vi "Distance Step Counter.vi"(8 "Distance (in)":dbl=40.0 format="%#_13g", 9 "Base Step":i32, 10 "Step":i32, 11 "RobotDriveDevRef":T1) -> (1 "Progress":dbl, 2 "Finished?":bool, 3 "Step out":i32)   [LabVIEW 2016]
uses:
  <vilib>/Rock Robotics/WPI/RobotDrive/WPI_RobotDriveDevRef.ctl
  <vilib>/Rock Robotics/WPI/MotorControl/WPI_MotorControlDeviceRef.ctl
  <vilib>/Rock Robotics/WPI/MotorControl/WPI_MotorControlType.ctl
  <vilib>/Rock Robotics/SystemInterfaces/DIO/FPGA_DIOPWMChannel.ctl
  <vilib>/Rock Robotics/WPI/PWM/WPI_PWMDeadband.ctl
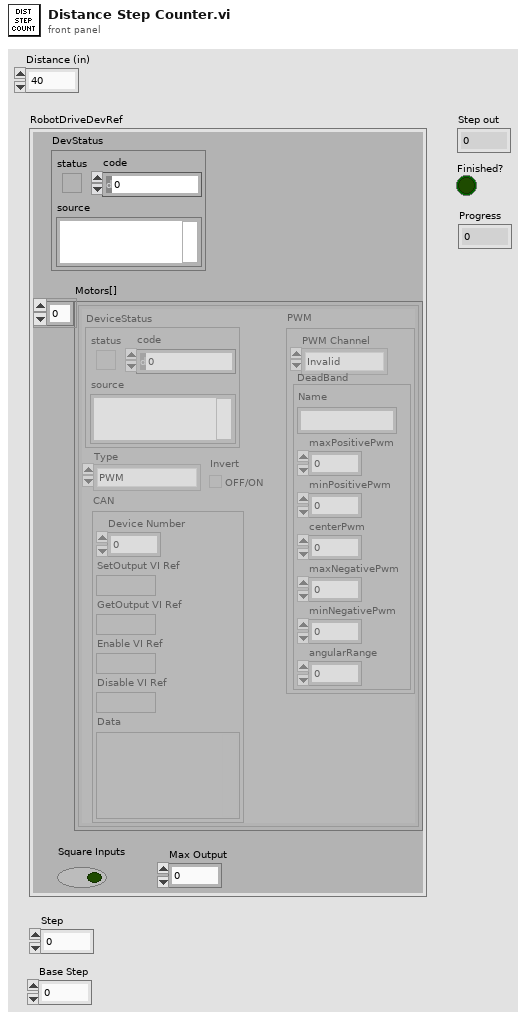
[diagram p1: front panel]
types:
  T1 = typedef "WPI_RobotDriveDevRef.ctl" = cluster{"DevStatus":errorcluster, "Motors[]":T2[], "Square Inputs":bool, "Max Output":dbl}
  T2 = typedef "WPI_MotorControlDeviceRef.ctl" = cluster{"DeviceStatus":errorcluster, "Type":T3, "PWM":cluster{"PWM Channel":T4, "DeadBand":T5}, "CAN":cluster{"Device Number":u8, "SetOutput VI Ref":variant, "GetOutput VI Ref":variant, "Enable VI Ref":variant, "Disable VI Ref":variant, "Data":variant}, "Invert":bool}
  T3 = typedef "WPI_MotorControlType.ctl" = enum16{"PWM", "CAN"}
  T4 = typedef "FPGA_DIOPWMChannel.ctl" = enum8{"PWM 0", "PWM 1", "PWM 2", "PWM 3", "PWM 4", "PWM 5", "PWM 6", "PWM 7", "PWM 8", "PWM 9", "PWM MXP 0", "PWM MXP 1", "PWM MXP 2", "PWM MXP 3", "PWM MXP 4", "PWM MXP 5", "PWM MXP 6", "PWM MXP 7", "PWM MXP 8", "PWM MXP 9", "Invalid"}
  T5 = typedef "WPI_PWMDeadband.ctl" = cluster{"Name":string, "maxPositivePwm":i32, "minPositivePwm":i32, "centerPwm":i32, "maxNegativePwm":i32, "minNegativePwm":i32, "angularRange":u16}
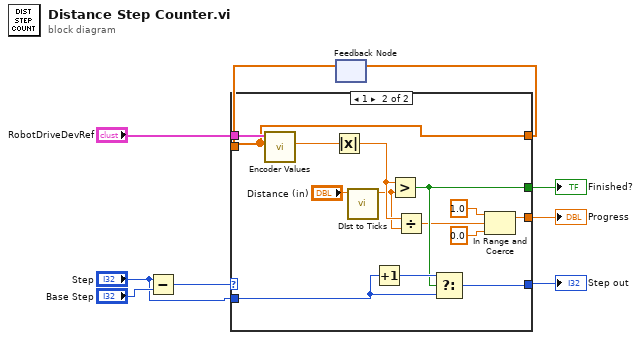
[diagram p0: block diagram]
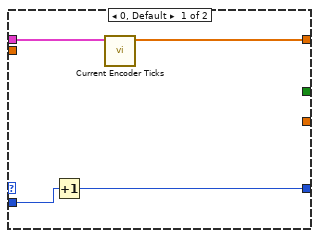
[diagram p2: hidden frame]
diagram:
  n1 = Subtract(x="Step", y="Base Step") -> (x-y=w5:i32)
  n2 = feedback #1() -> (w9:dbl[])  [unwired: 1 in]
  n3 = case shown="1" w5 {
    tunnel: "RobotDriveDevRef" -> [w12 w27]
    tunnel: [w13 w26] -> w7
    tunnel: [w11 w24] -> w8
    tunnel: w9 -> [_ w24]
    tunnel: [_ w21] -> w4
    tunnel: [_ w17] -> w3
    tunnel: "Step" -> [w10 w14]
    frame 0, Default {
      n4 = Increment(x=w10) -> (x+1=w13:i32)
      n5 = call "Current Encoder Ticks.vi"("RobotDriveDevRef"=w12) -> ("Array"=w11:dbl[])  [unwired: 10 in]
    }
    frame 1 {
      n6 = call "Encoder Values.vi"("Array"=w24, "RobotDriveDevRef"=w27) -> ("Position"=w23:dbl)  [unwired: 8 in, 1 out]
      n7 = Absolute Value(x=w23) -> (abs(x)=w20:dbl)
      n8 = call "DIst to Ticks.vi"("x"="Distance (in)") -> ("Numeric"=w19:dbl)  [unwired: 10 in]
      n9 = Increment(x=w14) -> (x+1=w25:i32)
      n10 = Greater?(x=w20, y=w19) -> (0:w21:bool)
      n11 = Divide(x=w20, y=w19) -> (x/y=w18:dbl)
      n12 = Select(t=w25, s=w21, f=w14) -> (s? t:f=w26:i32)
      n13 = In Range and Coerce(upper limit=1.0, x=w18, lower limit=0.0) -> (coerced(x)=w17:dbl)  [unwired: 1 out]
    }
  }
  "Step out" <- w7
  "Finished?" <- w4
  "Progress" <- w3
  n14 = feedback-in #1(w8) -> ()
